vi "获取量程参数存入关键参数.vi"(7 "关键参数变更":bool, 8 "error in (no error)":errorcluster caption="错误输入（无错误）", 9 "量程":u16, 10 "flowid":u16, 11 "id":u16) -> (0 "error out":errorcluster caption="错误输出")   [LabVIEW 2016, in "斯坦道通用流路CODmn.lvlib"]
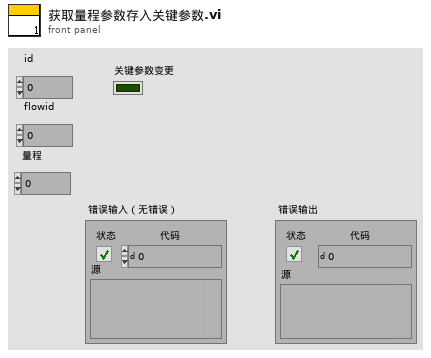
[diagram p1: front panel]
types:
  T1 = cluster{"运行模式":enum16{"维护模式", "常规模式", "应急模式", "质控模式"}, "质控频次":enum16{"关闭", "每天", "星期一", "星期二", "星期三", "星期四", "星期五", "星期六", "星期日"}, "空白核查时间":u16, "跨度核查时间":u16, "测量间隔":u16}
  T2 = cluster{"总磷":dbl, "总氮":dbl, "氨氮":dbl, "磷酸盐":dbl, "硝氮":dbl, "亚硝氮":dbl, "硅酸盐":dbl, "硫化物":dbl, "COD":dbl, "氟化物":dbl, "CODMn":dbl}
  T3 = cluster{"标液浓度1":dbl, "测量吸光度1":dbl, "样品1启用":bool, "标液浓度2":dbl, "测量吸光度2":dbl, "样品2启用":bool, "标液浓度3":dbl, "测量吸光度3":dbl, "样品3启用":bool, "标液浓度4":dbl, "测量吸光度4":dbl, "样品4启用":bool, "标液浓度5":dbl, "测量吸光度5":dbl, "样品5启用":bool, "模型":enum32{"线性", "多项式"}, "精度":dbl, "XY图":cluster{"X Values":dbl[], "Y Values":dbl[]}[], "拟合公式":string, "r^2":dbl, "标样一校准时间":timestamp, "标样二校准时间":timestamp, "标样三校准时间":timestamp, "标样四校准时间":timestamp, "标样五校准时间":timestamp, "二次方程":cluster{"c":dbl, "x":dbl, "x^2":dbl}, "标定时间":timestamp}
  T4 = cluster{"测量精度":u16, "检出限":dbl, "上限":dbl, "下限":dbl, "阈值（低->高）":dbl, "阈值（高->低）":dbl, "稀释度":dbl}
  T5 = typedef "斯坦道通用流路CODmn.lvlib/V3 A版外设参数.ctl" = cluster{"泵类型":u8, "进样速度":u32, "出样速度":u32, "泵阀量":u8, "阀方向":u8, "光谱仪类型":u8, "光谱采样次数":u8, "氙灯次数":u8, "B":u16, "C":u16, "D":u16, "E":u16, "B_COD":u16, "C_COD":u16, "D_COD":u16, "E_COD":u16, "G":u16, "M":u16, "N":u16, "氨氮注射泵控温下限":sgl, "氨氮注射泵控温上限":sgl, "总氮注射泵控温下限":sgl, "总氮注射泵控温上限":sgl, "消解温度下限":sgl, "消解温度上限":sgl, "加热10s限值":sgl, "KP":sgl, "KI":sgl, "KD":sgl, "高温高压阀开阀温度":sgl, "总氮x公式0":u8, "总氮x公式1":sgl, "总氮x公式2":sgl, "总磷浊度稀释系数":sgl, "总磷浊度补偿权重1":sgl, "总磷浊度补偿权重2":sgl, "盐度系数":sgl, "氨氮补偿系数1":sgl, "氨氮补偿系数2":sgl}
  T6 = cluster{"标液浓度1":dbl, "测量吸光度1":dbl, "样品1启用":bool, "标液浓度2":dbl, "测量吸光度2":dbl, "样品2启用":bool, "标液浓度3":dbl, "测量吸光度3":dbl, "样品3启用":bool, "标液浓度4":dbl, "测量吸光度4":dbl, "样品4启用":bool, "标液浓度5":dbl, "测量吸光度5":dbl, "样品5启用":bool, "模型":enum32{"线性", "多项式"}, "精度":dbl, "XY图":cluster{"X Values":dbl[], "Y Values":dbl[]}[], "拟合公式":string, "r^2":dbl, "标样一校准时间":timestamp, "标样二校准时间":timestamp, "标样三校准时间":timestamp, "标样四校准时间":timestamp, "标样五校准时间":timestamp, "二次方程":cluster{"c":dbl, "x":dbl, "x^2":dbl}, "标定时间":timestamp}[]
  T7 = typedef "斯坦道通用流路CODmn.lvlib/关键参数.ctl" = cluster{"测量量程":sgl, "测量检出限":sgl, "测量精度":sgl, "测量间隔":sgl, "消解温度":sgl, "消解时长":sgl, "三项式系数":sgl, "二次多项式系数":sgl, "曲线斜率":sgl, "曲线截距":sgl, "线性相关系数":sgl, "空白校准时间":timestamp, "标样校准时间":timestamp, "测量信号值":sgl, "稀释倍数":sgl, "空白标定系数":sgl, "量程系数":sgl}
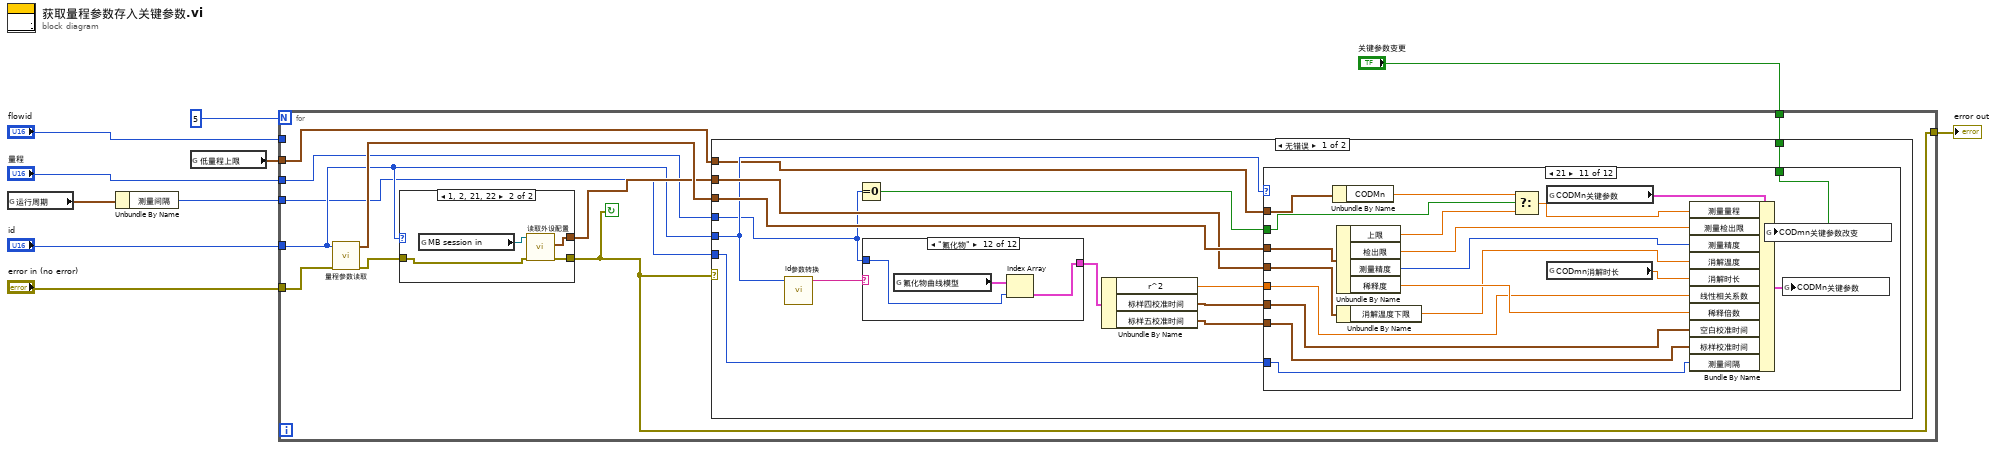
[diagram p0: block diagram]
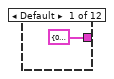
[diagram p3: hidden frame]
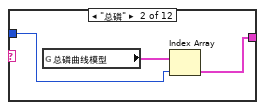
[diagram p4: hidden frame]
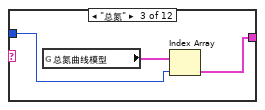
[diagram p5: hidden frame]
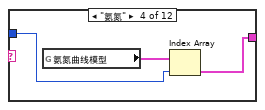
[diagram p6: hidden frame]
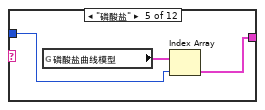
[diagram p7: hidden frame]
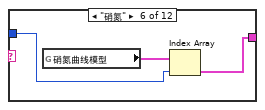
[diagram p8: hidden frame]
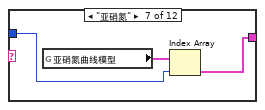
[diagram p9: hidden frame]
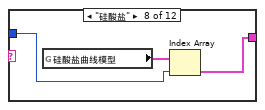
[diagram p10: hidden frame]
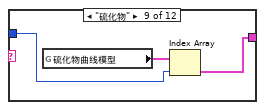
[diagram p11: hidden frame]
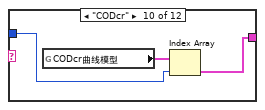
[diagram p12: hidden frame]
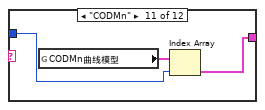
[diagram p13: hidden frame]
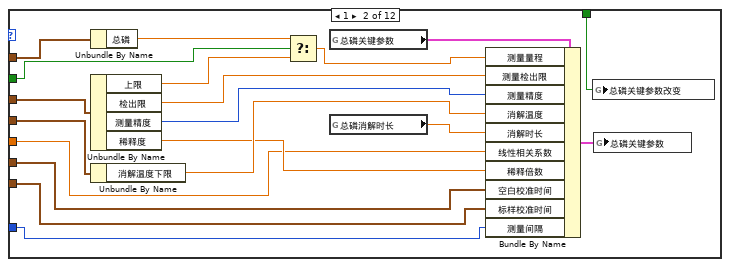
[diagram p15: hidden frame]
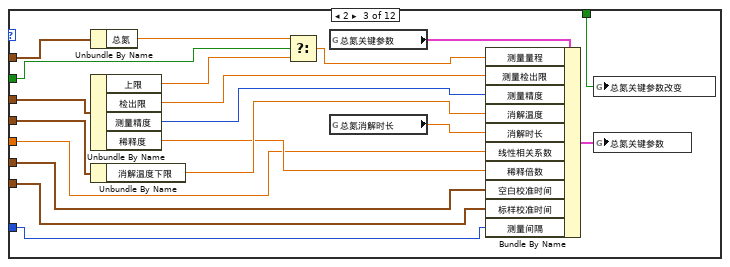
[diagram p16: hidden frame]
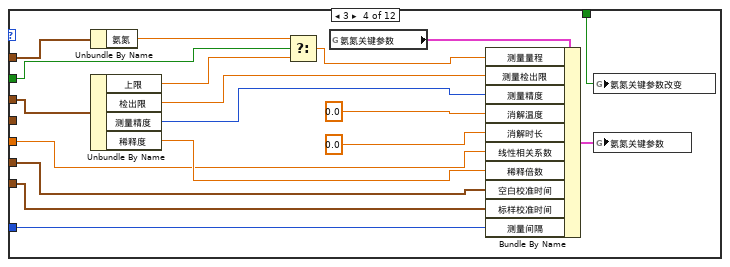
[diagram p17: hidden frame]
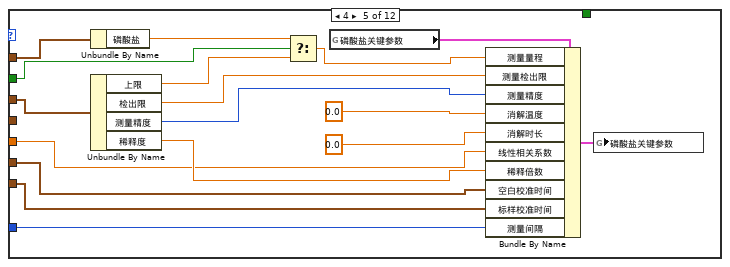
[diagram p18: hidden frame]
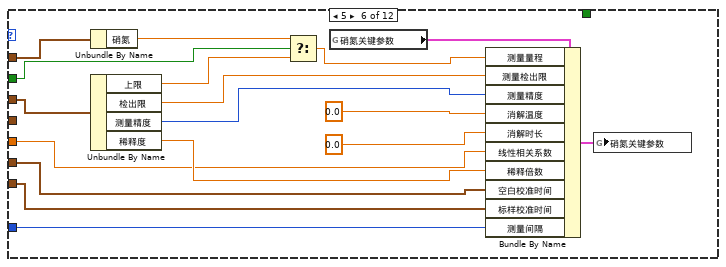
[diagram p19: hidden frame]
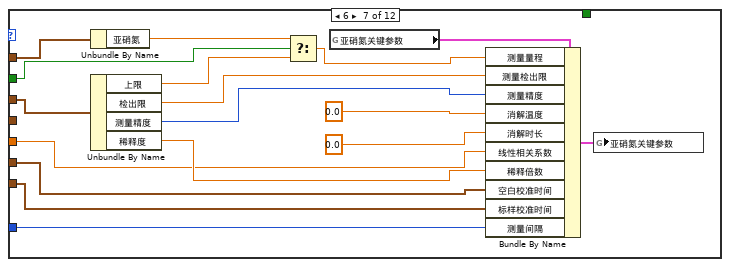
[diagram p20: hidden frame]
diagram:
  n1 = global read "总磷总氮断电保存全局变量.vi" "运行周期"() -> (w4:T1)
  n2 = Unbundle By Name(w4) -> ("测量间隔"=w3:u16)
  n3 = global read "总磷总氮断电保存全局变量.vi" "低量程上限"() -> (w2:T2)
  n4 = for {
    N: 5 -> [_]
    tunnel: "量程" -> [w18]
    tunnel: "flowid" -> [_]
    tunnel: "id" -> [w14]
    tunnel: "error in (no error)" -> [w15]
    tunnel: [w16] -> w5
    tunnel: w3 -> [w13]
    tunnel: w2 -> [w12]
    tunnel: "关键参数变更" -> [w11]
    stop <- w16 continue-if-true
    n5 = call "量程参数读取.vi"("error in (no error)"=w15, "测量参数"=w14) -> ("error out"=w17:errorcluster, "量程参数读取"=w20:T4)  [unwired: 8 in]
    n6 = case shown="1, 2, 21, 22" w14 {
      tunnel: [_ w24] -> w19
      tunnel: w17 -> [w21 w23]
      tunnel: [w21 w22] -> w16
      frame 0, Default {
      }
      frame 1, 2, 21, 22 {
        n7 = global read "VAR总磷总氮全局变量.vi" "MB session in"() -> (w25:refnum<class "MB_Master.lvclass">)
        n8 = call "读取外设配置.vi"("error in (no error)"=w23, "MB session in"=w25) -> ("error out"=w22:errorcluster, "外设配置"=w24:T5)  [unwired: 7 in, 1 out]
      }
    }
    n9 = case shown="无错误" w16 {
      tunnel: w20 -> [w38 _]
      tunnel: w19 -> [w37 _]
      tunnel: w14 -> [w31 _]
      tunnel: w18 -> [w28 _]
      tunnel: w13 -> [w30 _]
      tunnel: w12 -> [w29 _]
      tunnel: w11 -> [w26 _]
      frame No Error {
        n10 = call "id参数转换.vi"("id"=w31) -> ("table输出"=w36:string)  [unwired: 9 in, 1 out]
        n11 = Equal To 0?(x=w28) -> (x = 0?=w27:bool)
        n12 = case shown="\"氟化物\"" w36 {
          tunnel: w28 -> [_ w40 w43 w46 w49 w52 w55 w58 w61 w64 w67 w70]
          tunnel: [T3 {"标液浓度1"=0.0, "测量吸光度1"=0.0, "样品1启用"=FALSE, "标液浓度2"=0.0, "测量吸光度2"=0.0, "样品2启用"=FALSE, "标液浓度3"=0.0, "测量吸光度3"=0.0, "样品3启用"=FALSE, "标液浓度4"=0.0, "测量吸光度4"=0.0, "样品4启用"=FALSE, "标液浓度5"=0.0, "测量吸光度5"=0.0, "样品5启用"=FALSE, "模型"=enum."线性", "精度"=0.0, "XY图"=[], "拟合公式"="", "r^2"=0.0, "标样一校准时间"=timestamp(0 s since 1904-01-01), "标样二校准时间"=timestamp(0 s since 1904-01-01), "标样三校准时间"=timestamp(0 s since 1904-01-01), "标样四校准时间"=timestamp(0 s since 1904-01-01), "标样五校准时间"=timestamp(0 s since 1904-01-01), "二次方程"={"c"=0.0, "x"=0.0, "x^2"=0.0}, "标定时间"=timestamp(0 s since 1904-01-01)} ("总磷曲线模型") w41 w44 w47 w50 w53 w56 w59 w62 w65 w68 w71] -> w35
          frame Default {
          }
          frame "总磷" {
            n13 = global read "校准数据全局变量.vi" "总磷曲线模型"() -> (w42:T6)
            n14 = Index Array(array=w42, index=w40) -> (element=w41:T3)
          }
          frame "总氮" {
            n15 = global read "校准数据全局变量.vi" "总氮曲线模型"() -> (w45:T6)
            n16 = Index Array(array=w45, index=w43) -> (element=w44:T3)
          }
          frame "氨氮" {
            n17 = global read "校准数据全局变量.vi" "氨氮曲线模型"() -> (w48:T6)
            n18 = Index Array(array=w48, index=w46) -> (element=w47:T3)
          }
          frame "磷酸盐" {
            n19 = global read "校准数据全局变量.vi" "磷酸盐曲线模型"() -> (w51:T6)
            n20 = Index Array(array=w51, index=w49) -> (element=w50:T3)
          }
          frame "硝氮" {
            n21 = global read "校准数据全局变量.vi" "硝氮曲线模型"() -> (w54:T6)
            n22 = Index Array(array=w54, index=w52) -> (element=w53:T3)
          }
          frame "亚硝氮" {
            n23 = global read "校准数据全局变量.vi" "亚硝氮曲线模型"() -> (w57:T6)
            n24 = Index Array(array=w57, index=w55) -> (element=w56:T3)
          }
          frame "硅酸盐" {
            n25 = global read "校准数据全局变量.vi" "硅酸盐曲线模型"() -> (w60:T6)
            n26 = Index Array(array=w60, index=w58) -> (element=w59:T3)
          }
          frame "硫化物" {
            n27 = global read "校准数据全局变量.vi" "硫化物曲线模型"() -> (w63:T6)
            n28 = Index Array(array=w63, index=w61) -> (element=w62:T3)
          }
          frame "CODcr" {
            n29 = global read "校准数据全局变量.vi" "CODcr曲线模型"() -> (w66:T6)
            n30 = Index Array(array=w66, index=w64) -> (element=w65:T3)
          }
          frame "CODMn" {
            n31 = global read "校准数据全局变量.vi" "CODMn曲线模型"() -> (w69:T6)
            n32 = Index Array(array=w69, index=w67) -> (element=w68:T3)
          }
          frame "氟化物" {
            n33 = global read "校准数据全局变量.vi" "氟化物曲线模型"() -> (w72:T6)
            n34 = Index Array(array=w72, index=w70) -> (element=w71:T3)
          }
        }
        n35 = Unbundle By Name(w35) -> ("r^2"=w34:dbl, "标样四校准时间"=w33:timestamp, "标样五校准时间"=w32:timestamp)
        n36 = case shown="21" w31 {
          tunnel: w38 -> [_ w89 w108 w126 w143 w160 w177 w194 w211 w230 w249 w267]
          tunnel: w37 -> [_ w86 w105 _ _ _ _ _ _ w226 w245 w263]
          tunnel: w34 -> [_ w80 w101 w120 w135 w154 w171 w188 w203 w223 w242 w260]
          tunnel: w33 -> [_ w81 w100 w119 w137 w153 w170 w187 w205 w222 w241 w259]
          tunnel: w32 -> [_ w82 w99 w118 w136 w152 w169 w186 w204 w221 w240 w258]
          tunnel: w30 -> [_ w79 w98 w117 w134 w151 w168 w185 w202 w220 w239 w257]
          tunnel: w29 -> [_ w78 w96 w115 w132 w149 w166 w182 w200 w218 w237 w255]
          tunnel: w27 -> [_ w76 w95 w114 w131 w148 w165 w183 w199 w217 w236 w254]
          tunnel: w26 -> [_ w73 w92 w111 _ _ _ _ _ w214 w233 _]
          frame 0, Default {
          }
          frame 1 {
            n37 = Unbundle By Name(w78) -> ("总磷"=w77:dbl)
            n38 = Unbundle By Name(w89) -> ("上限"=w75:dbl, "检出限"=w88:dbl, "测量精度"=w87:u16, "稀释度"=w83:dbl)
            n39 = Unbundle By Name(w86) -> ("消解温度下限"=w85:sgl)
            n40 = Select(t=w77, s=w76, f=w75) -> (s? t:f=w74:dbl)
            n41 = global read "VAR总磷总氮全局变量.vi" "总磷关键参数"() -> (w90:T7)
            n42 = global read "总磷总氮断电保存全局变量.vi" "总磷消解时长"() -> (w84:dbl)
            n43 = Bundle By Name(cluster=w90, "测量量程"=w74, "测量检出限"=w88, "测量精度"=w87, "消解温度"=w85, "消解时长"=w84, "线性相关系数"=w80, "稀释倍数"=w83, "空白校准时间"=w81, "标样校准时间"=w82, "测量间隔"=w79) -> (w91:T7)
            n44 = global write "VAR总磷总氮全局变量.vi" "总磷关键参数改变"(w73) -> ()
            n45 = global write "VAR总磷总氮全局变量.vi" "总磷关键参数"(w91) -> ()
          }
          frame 2 {
            n46 = Unbundle By Name(w96) -> ("总氮"=w97:dbl)
            n47 = Unbundle By Name(w108) -> ("上限"=w94:dbl, "检出限"=w107:dbl, "测量精度"=w106:u16, "稀释度"=w102:dbl)
            n48 = Unbundle By Name(w105) -> ("消解温度下限"=w104:sgl)
            n49 = Select(t=w97, s=w95, f=w94) -> (s? t:f=w93:dbl)
            n50 = global read "VAR总磷总氮全局变量.vi" "总氮关键参数"() -> (w109:T7)
            n51 = global read "总磷总氮断电保存全局变量.vi" "总氮消解时长"() -> (w103:dbl)
            n52 = Bundle By Name(cluster=w109, "测量量程"=w93, "测量检出限"=w107, "测量精度"=w106, "消解温度"=w104, "消解时长"=w103, "线性相关系数"=w101, "稀释倍数"=w102, "空白校准时间"=w100, "标样校准时间"=w99, "测量间隔"=w98) -> (w110:T7)
            n53 = global write "VAR总磷总氮全局变量.vi" "总氮关键参数改变"(w92) -> ()
            n54 = global write "VAR总磷总氮全局变量.vi" "总氮关键参数"(w110) -> ()
          }
          frame 3 {
            n55 = Unbundle By Name(w115) -> ("氨氮"=w116:dbl)
            n56 = Unbundle By Name(w126) -> ("上限"=w113:dbl, "检出限"=w125:dbl, "测量精度"=w124:u16, "稀释度"=w123:dbl)
            n57 = Select(t=w116, s=w114, f=w113) -> (s? t:f=w112:dbl)
            n58 = global read "VAR总磷总氮全局变量.vi" "氨氮关键参数"() -> (w127:T7)
            n59 = Bundle By Name(cluster=w127, "测量量程"=w112, "测量检出限"=w125, "测量精度"=w124, "消解温度"=sgl 0.0, "消解时长"=sgl 0.0, "线性相关系数"=w120, "稀释倍数"=w123, "空白校准时间"=w119, "标样校准时间"=w118, "测量间隔"=w117) -> (w128:T7)
            n60 = global write "VAR总磷总氮全局变量.vi" "氨氮关键参数改变"(w111) -> ()
            n61 = global write "VAR总磷总氮全局变量.vi" "氨氮关键参数"(w128) -> ()
          }
          frame 4 {
            n62 = Unbundle By Name(w132) -> ("磷酸盐"=w133:dbl)
            n63 = Unbundle By Name(w143) -> ("上限"=w130:dbl, "检出限"=w142:dbl, "测量精度"=w141:u16, "稀释度"=w140:dbl)
            n64 = Select(t=w133, s=w131, f=w130) -> (s? t:f=w129:dbl)
            n65 = global read "VAR总磷总氮全局变量.vi" "磷酸盐关键参数"() -> (w144:T7)
            n66 = Bundle By Name(cluster=w144, "测量量程"=w129, "测量检出限"=w142, "测量精度"=w141, "消解温度"=sgl 0.0, "消解时长"=sgl 0.0, "线性相关系数"=w135, "稀释倍数"=w140, "空白校准时间"=w137, "标样校准时间"=w136, "测量间隔"=w134) -> (w145:T7)
            n67 = global write "VAR总磷总氮全局变量.vi" "磷酸盐关键参数"(w145) -> ()
          }
          frame 5 {
            n68 = Unbundle By Name(w149) -> ("硝氮"=w150:dbl)
            n69 = Unbundle By Name(w160) -> ("上限"=w147:dbl, "检出限"=w159:dbl, "测量精度"=w158:u16, "稀释度"=w157:dbl)
            n70 = Select(t=w150, s=w148, f=w147) -> (s? t:f=w146:dbl)
            n71 = global read "VAR总磷总氮全局变量.vi" "硝氮关键参数"() -> (w161:T7)
            n72 = Bundle By Name(cluster=w161, "测量量程"=w146, "测量检出限"=w159, "测量精度"=w158, "消解温度"=sgl 0.0, "消解时长"=sgl 0.0, "线性相关系数"=w154, "稀释倍数"=w157, "空白校准时间"=w153, "标样校准时间"=w152, "测量间隔"=w151) -> (w162:T7)
            n73 = global write "VAR总磷总氮全局变量.vi" "硝氮关键参数"(w162) -> ()
          }
          frame 6 {
            n74 = Unbundle By Name(w166) -> ("亚硝氮"=w167:dbl)
            n75 = Unbundle By Name(w177) -> ("上限"=w164:dbl, "检出限"=w176:dbl, "测量精度"=w175:u16, "稀释度"=w174:dbl)
            n76 = Select(t=w167, s=w165, f=w164) -> (s? t:f=w163:dbl)
            n77 = global read "VAR总磷总氮全局变量.vi" "亚硝氮关键参数"() -> (w178:T7)
            n78 = Bundle By Name(cluster=w178, "测量量程"=w163, "测量检出限"=w176, "测量精度"=w175, "消解温度"=sgl 0.0, "消解时长"=sgl 0.0, "线性相关系数"=w171, "稀释倍数"=w174, "空白校准时间"=w170, "标样校准时间"=w169, "测量间隔"=w168) -> (w179:T7)
            n79 = global write "VAR总磷总氮全局变量.vi" "亚硝氮关键参数"(w179) -> ()
          }
          frame 7 {
            n80 = Unbundle By Name(w182) -> ("硅酸盐"=w184:dbl)
            n81 = Unbundle By Name(w194) -> ("上限"=w181:dbl, "检出限"=w193:dbl, "测量精度"=w192:u16, "稀释度"=w191:dbl)
            n82 = Select(t=w184, s=w183, f=w181) -> (s? t:f=w180:dbl)
            n83 = global read "VAR总磷总氮全局变量.vi" "硅酸盐关键参数"() -> (w195:T7)
            n84 = Bundle By Name(cluster=w195, "测量量程"=w180, "测量检出限"=w193, "测量精度"=w192, "消解温度"=sgl 0.0, "消解时长"=sgl 0.0, "线性相关系数"=w188, "稀释倍数"=w191, "空白校准时间"=w187, "标样校准时间"=w186, "测量间隔"=w185) -> (w196:T7)
            n85 = global write "VAR总磷总氮全局变量.vi" "硅酸盐关键参数"(w196) -> ()
          }
          frame 8 {
            n86 = Unbundle By Name(w200) -> ("硫化物"=w201:dbl)
            n87 = Unbundle By Name(w211) -> ("上限"=w198:dbl, "检出限"=w210:dbl, "测量精度"=w209:u16, "稀释度"=w208:dbl)
            n88 = Select(t=w201, s=w199, f=w198) -> (s? t:f=w197:dbl)
            n89 = global read "VAR总磷总氮全局变量.vi" "硫化物关键参数"() -> (w212:T7)
            n90 = Bundle By Name(cluster=w212, "测量量程"=w197, "测量检出限"=w210, "测量精度"=w209, "消解温度"=sgl 0.0, "消解时长"=sgl 0.0, "线性相关系数"=w203, "稀释倍数"=w208, "空白校准时间"=w205, "标样校准时间"=w204, "测量间隔"=w202) -> (w213:T7)
            n91 = global write "VAR总磷总氮全局变量.vi" "硫化物关键参数"(w213) -> ()
          }
          frame 22 {
            n92 = Unbundle By Name(w218) -> ("亚硝氮"=w219:dbl)
            n93 = Unbundle By Name(w230) -> ("上限"=w216:dbl, "检出限"=w229:dbl, "测量精度"=w228:u16, "稀释度"=w227:dbl)
            n94 = Unbundle By Name(w226) -> ("消解温度下限"=w225:sgl)
            n95 = Select(t=w219, s=w217, f=w216) -> (s? t:f=w215:dbl)
            n96 = global read "VAR总磷总氮全局变量.vi" "CODcr关键参数"() -> (w231:T7)
            n97 = global read "总磷总氮断电保存全局变量.vi" "CODcr消解时长"() -> (w224:dbl)
            n98 = Bundle By Name(cluster=w231, "测量量程"=w215, "测量检出限"=w229, "测量精度"=w228, "消解温度"=w225, "消解时长"=w224, "线性相关系数"=w223, "稀释倍数"=w227, "空白校准时间"=w222, "标样校准时间"=w221, "测量间隔"=w220) -> (w232:T7)
            n99 = global write "VAR总磷总氮全局变量.vi" "CODCr关键参数改变"(w214) -> ()
            n100 = global write "VAR总磷总氮全局变量.vi" "CODcr关键参数"(w232) -> ()
          }
          frame 21 {
            n101 = Unbundle By Name(w237) -> ("CODMn"=w238:dbl)
            n102 = Unbundle By Name(w249) -> ("上限"=w235:dbl, "检出限"=w248:dbl, "测量精度"=w247:u16, "稀释度"=w246:dbl)
            n103 = Unbundle By Name(w245) -> ("消解温度下限"=w244:sgl)
            n104 = Select(t=w238, s=w236, f=w235) -> (s? t:f=w234:dbl)
            n105 = global read "VAR总磷总氮全局变量.vi" "CODMn关键参数"() -> (w250:T7)
            n106 = global read "总磷总氮断电保存全局变量.vi" "CODmn消解时长"() -> (w243:dbl)
            n107 = Bundle By Name(cluster=w250, "测量量程"=w234, "测量检出限"=w248, "测量精度"=w247, "消解温度"=w244, "消解时长"=w243, "线性相关系数"=w242, "稀释倍数"=w246, "空白校准时间"=w241, "标样校准时间"=w240, "测量间隔"=w239) -> (w251:T7)
            n108 = global write "VAR总磷总氮全局变量.vi" "CODmn关键参数改变"(w233) -> ()
            n109 = global write "VAR总磷总氮全局变量.vi" "CODMn关键参数"(w251) -> ()
          }
          frame 50 {
            n110 = Unbundle By Name(w255) -> ("氟化物"=w256:dbl)
            n111 = Unbundle By Name(w267) -> ("上限"=w253:dbl, "检出限"=w266:dbl, "测量精度"=w265:u16, "稀释度"=w264:dbl)
            n112 = Unbundle By Name(w263) -> ("消解温度下限"=w262:sgl)
            n113 = Select(t=w256, s=w254, f=w253) -> (s? t:f=w252:dbl)
            n114 = global read "总磷总氮断电保存全局变量.vi" "CODmn消解时长"() -> (w261:dbl)
            n115 = global read "VAR总磷总氮全局变量.vi" "氟化物关键参数"() -> (w268:T7)
            n116 = Bundle By Name(cluster=w268, "测量量程"=w252, "测量检出限"=w266, "测量精度"=w265, "消解温度"=w262, "消解时长"=w261, "线性相关系数"=w260, "稀释倍数"=w264, "空白校准时间"=w259, "标样校准时间"=w258, "测量间隔"=w257) -> (w269:T7)
            n117 = global write "VAR总磷总氮全局变量.vi" "氟化物关键参数"(w269) -> ()
          }
        }
      }
      frame Error {
      }
    }
  }
  "error out" <- w5
